vi "RSA New.vi"(8 "error in (no error)":errorcluster, 11 "KeySize (384 .. 16384)":i32=384 min=384 max=16384 step=8) -> (0 "error out":errorcluster, 3 "RSA out":refnum<class "RSA.lvclass">)   [LabVIEW 2021, in "RSA.lvclass"]
uses:
  RSA.lvclass
  RSA.lvclass/RSA.ctl
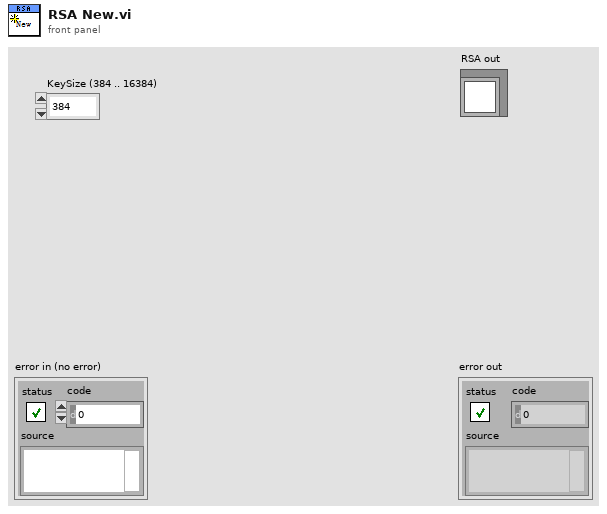
[diagram p1: front panel]
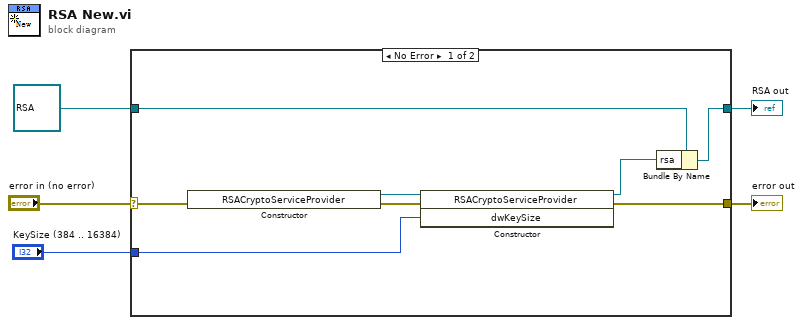
[diagram p0: block diagram]
diagram:
  n1 = case shown="No Error" "error in (no error)" {
    selector: "error in (no error)" -> [w10 w15]
    tunnel: [w11 w15] -> w4
    tunnel: [w12 w14] -> w2
    tunnel: refnum<class "RSA.lvclass"> refnum ("RSA in") -> [w6 w14]
    tunnel: "KeySize (384 .. 16384)" -> [w13 _]
    frame No Error {
      n2 = constructor class="RSACryptoServiceProvider" ("AliceEntschlüsselt")(error in=w10) -> (reference out=w8:refnum<k24>, error out=w9:errorcluster)  [unwired: 2 in, 1 out]
      n3 = constructor class="RSACryptoServiceProvider" ("AliceErstelltPrivateKeyUndPublicKey")(reference=w8, error in=w9, "dwKeySize"=w13) -> (reference out=w7:refnum<k24>, error out=w11:errorcluster)  [unwired: 1 in, 2 out]
      n4 = Bundle By Name(cluster=w6, "rsa"=w7) -> (w12:refnum<class "RSA.lvclass">)
    }
    frame Error {
    }
  }
  "error out" <- w4
  "RSA out" <- w2
